vi "plot theory.vi"() -> ()   [LabVIEW 2016]
uses:
  <vilib>/Utility/file.llb/Write Delimited Spreadsheet (DBL).vi
  <userlib>/LevyLab/Graph Utilities/graph_utilities.lvclass
panel:
  in  "color scale":u32[](array[colorbox])=[16711680, 16772608, 6618880, 3381759, 16860, 10420479]
  in  "length 2":i32=200
  in  "index 2":i32
  out "Intensity Graph 13":dbl[][](graph)
  in  "file path (dialog if empty)":path=path "C:/Users/ansom/OneDrive/Pascal Electron Bunching/Figures/Fig 4_new/DMRG stuff/trion_from labview.txt"
  out "Array 2":dbl[][](array[numeric])
  in  "DMRG #":i32=226
  in  "file (use dialog) 4":path=path "C:/Users/ansom/OneDrive/Pascal Electron Bunching/Figures/Fig 4_new/DMRG stuff/trion.txt"
  in  "length":i32=1000
  in  "index":i32
  out "input G":cluster{dbl[], dbl[]}[](graph)
  in  "mu":path=path "C:/Users/ansom/OneDrive/Pascal Electron Bunching/Figures/Fig 3_new/mathematica/mu.txt"
  in  "G":path=path "C:/Users/ansom/OneDrive/Pascal Electron Bunching/Figures/Fig 3_new/mathematica/Gsteps_g=1"
  in  "Numeric 2":i32=100
  in  "Numeric":i32=360
  out "Intensity Graph 12":dbl[][](graph)
  out "Array":dbl[][](array[numeric])
  in  "file (use dialog)":path=path "C:/Users/ansom/OneDrive/Pascal Electron Bunching/Figures/Fig 3_new/mathematica/ModeldGdE"
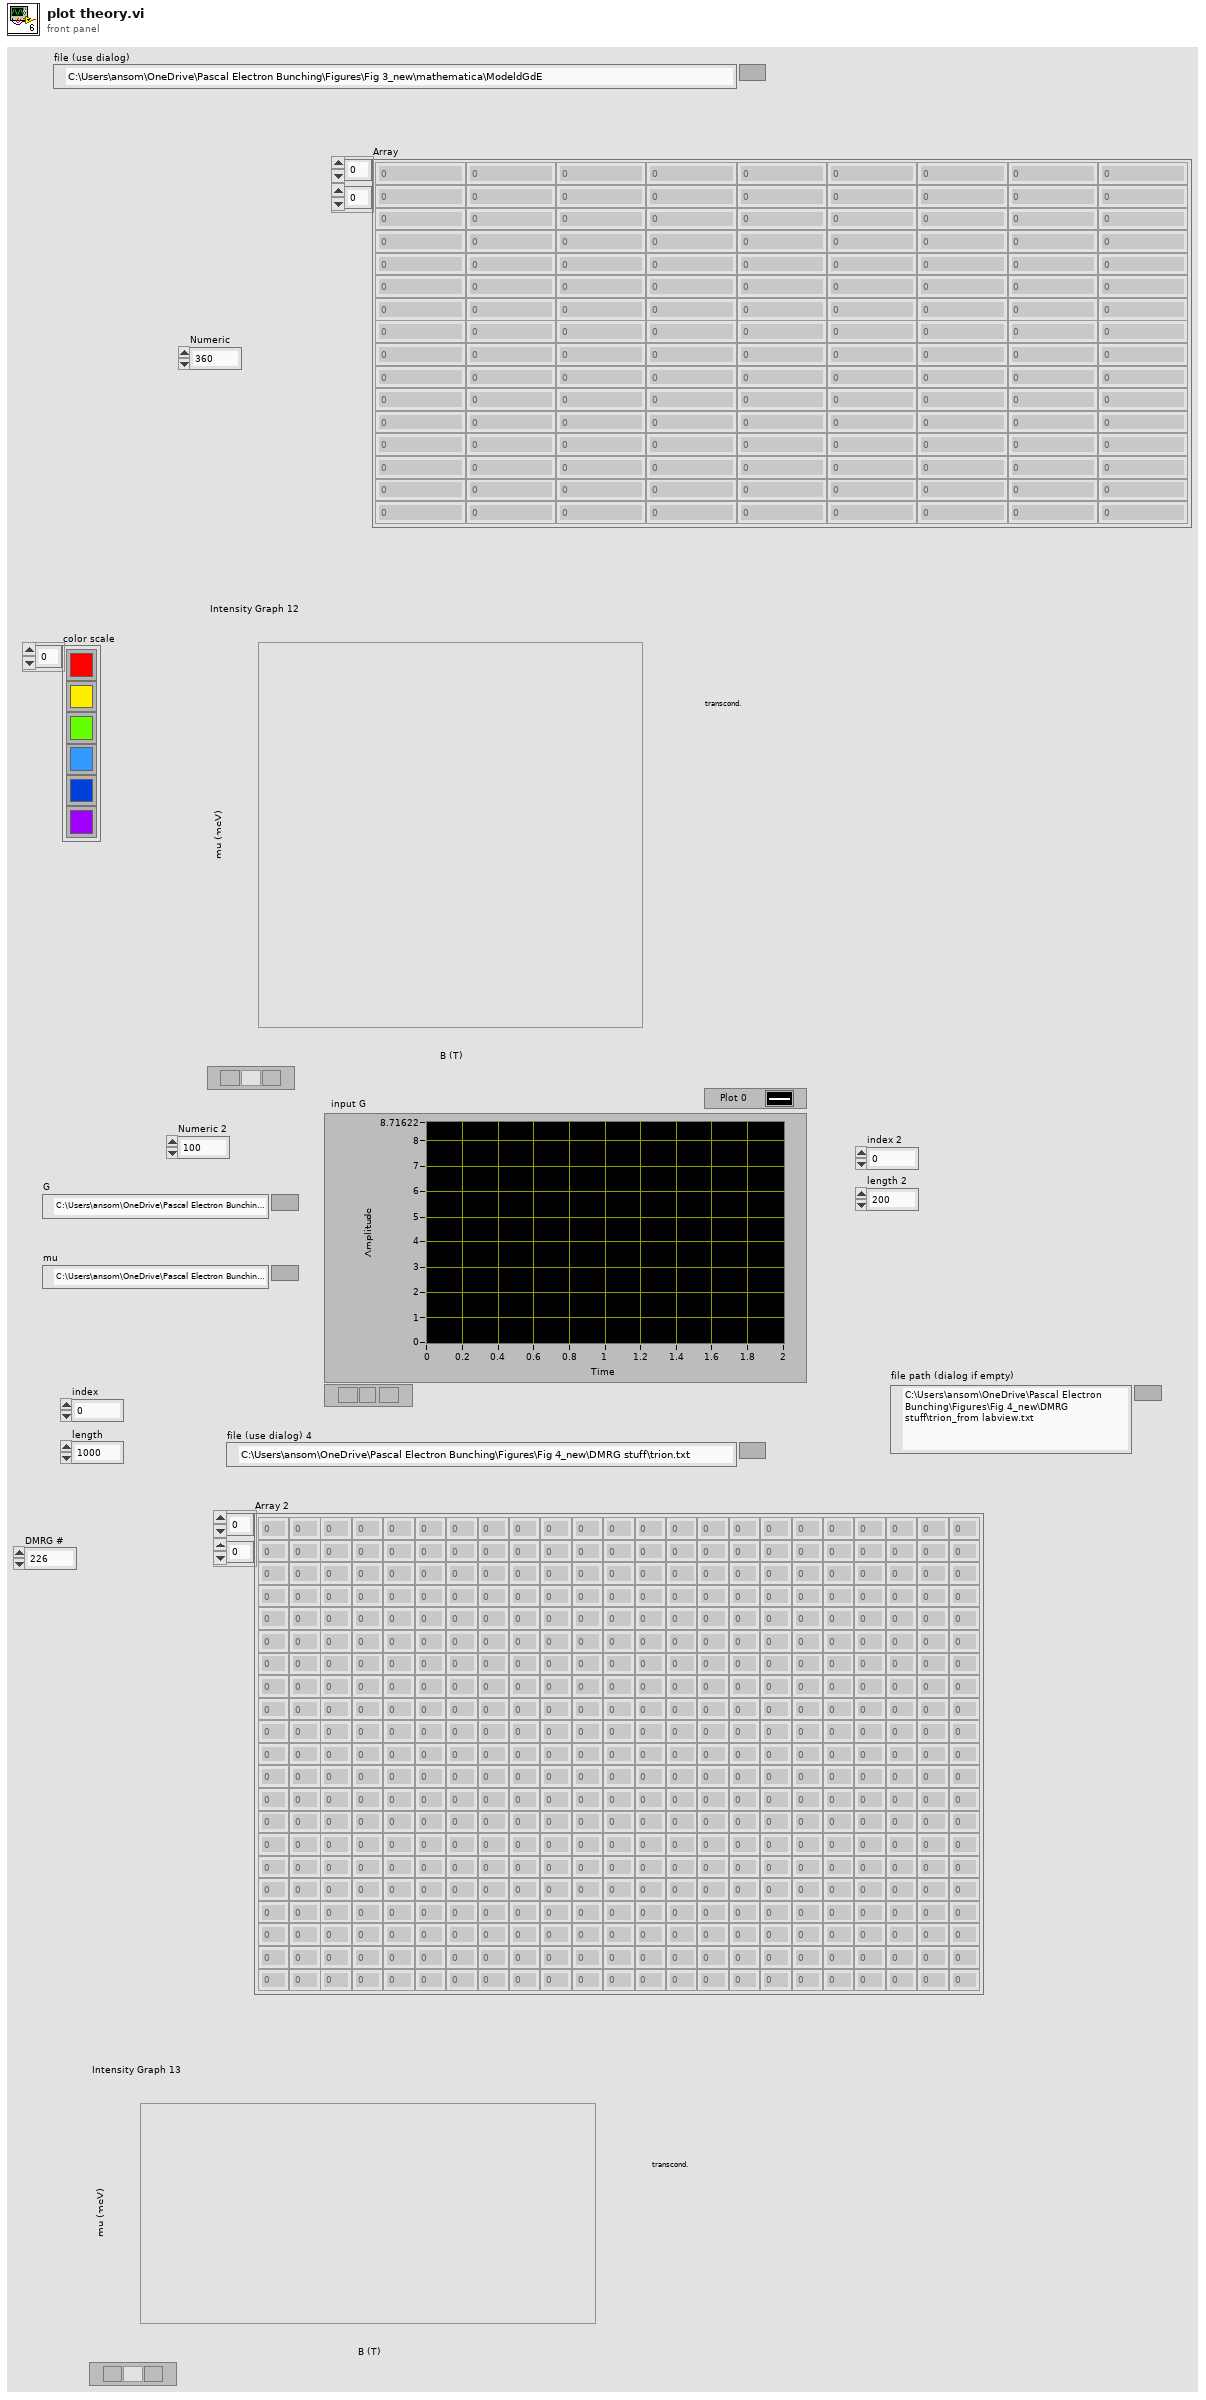
[diagram p1: front panel]
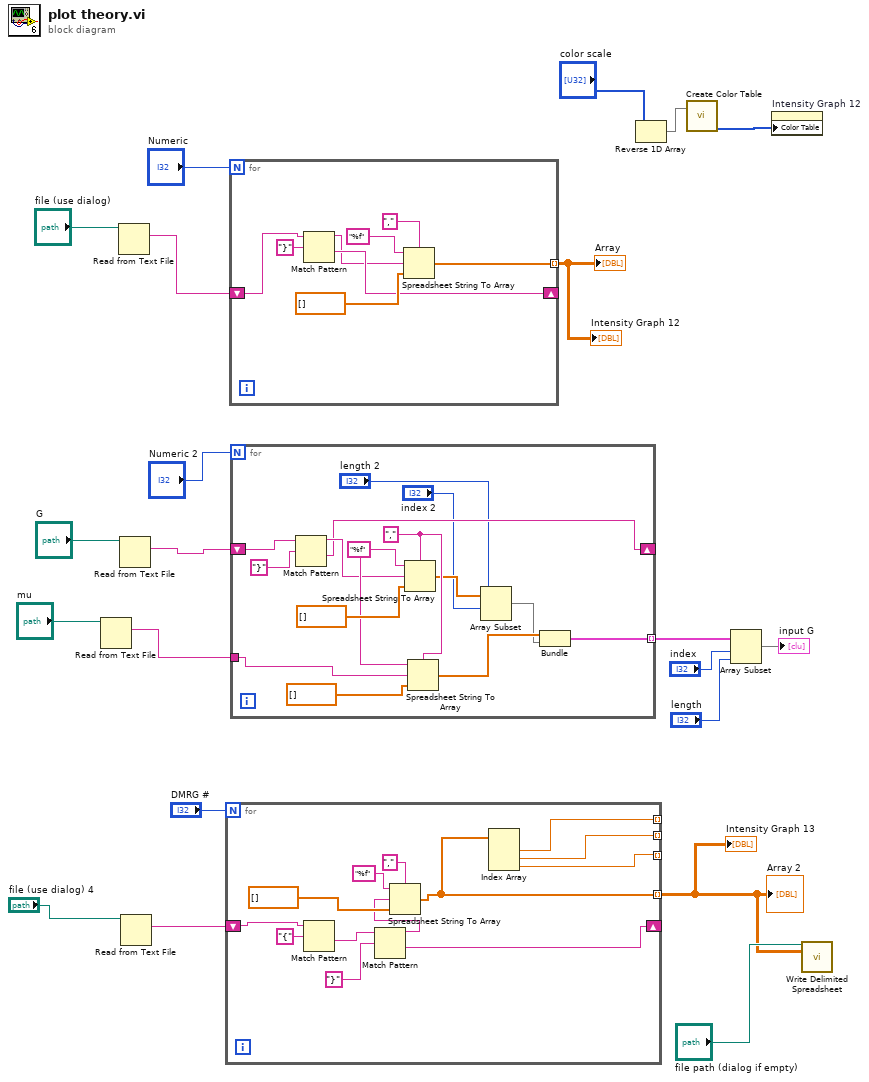
[diagram p0: block diagram]
diagram:
  n1 = Read from Text File(file (use dialog)="mu") -> (text=w14:string)  [unwired: 3 in, 3 out]
  n2 = Read from Text File(file (use dialog)="file (use dialog)") -> (text=w20:string)  [unwired: 3 in, 3 out]
  n3 = Read from Text File(file (use dialog)="G") -> (text=w13:string)  [unwired: 3 in, 3 out]
  n4 = Read from Text File(file (use dialog)="file (use dialog) 4") -> (text=w7:string)  [unwired: 3 in, 3 out]
  n5 = for {
    N: "DMRG #" -> [_]
    shift-right: [w26] -> _
    shift-left: w7 -> [w33]
    tunnel: [w25] -> w4 mode=indexing
    tunnel: [w24] -> _ mode=indexing
    tunnel: [w23] -> _ mode=indexing
    tunnel: [w22] -> _ mode=indexing
    n6 = Match Pattern(string=w33, regular expression="{") -> (after substring=w29:string)  [unwired: 1 in, 3 out]
    n7 = Match Pattern(string=w29, regular expression="}") -> (before substring=w27:string, after substring=w26:string)  [unwired: 1 in, 2 out]
    n8 = Spreadsheet String To Array(delimiter (Tab)=",", format string="%f", spreadsheet string=w27, array type (2D Dbl)=dbl[] []) -> (array=w25:dbl[])
    n9 = Index Array(array=w25) -> (element #1=w24:dbl, element #2=w23:dbl, element #3=w22:dbl)  [unwired: 3 in]
  }
  "Array 2" <- w4
  "Intensity Graph 13" <- w4
  n10 = for {
    N: "Numeric" -> [_]
    tunnel: [w38] -> w18 mode=indexing
    shift-right: [w37] -> _
    shift-left: w20 -> [w36]
    n11 = Match Pattern(string=w36, regular expression="}") -> (before substring=w35:string, after substring=w37:string)  [unwired: 1 in, 2 out]
    n12 = Spreadsheet String To Array(delimiter (Tab)=",", format string="%f", spreadsheet string=w35, array type (2D Dbl)=dbl[] []) -> (array=w38:dbl[])
  }
  "Array" <- w18
  "Intensity Graph 12" <- w18
  n13 = for {
    N: "Numeric 2" -> [_]
    tunnel: w14 -> [w56]
    tunnel: [w52] -> w12 mode=indexing
    shift-right: [w48] -> _
    shift-left: w13 -> [w51]
    w55 = "%f" ("format string")
    w54 = "," ("delimiter (Tab)")
    n14 = Match Pattern(string=w51, regular expression="}") -> (before substring=w49:string, after substring=w48:string)  [unwired: 1 in, 2 out]
    n15 = Spreadsheet String To Array(delimiter (Tab)=w54, format string=w55, spreadsheet string=w49, array type (2D Dbl)=dbl[] []) -> (array=w46:dbl[])
    n16 = Spreadsheet String To Array(delimiter (Tab)=w54, format string=w55, spreadsheet string=w56, array type (2D Dbl)=dbl[] []) -> (array=w47:dbl[])
    n17 = Array Subset(array=w46, index="index 2", length="length 2") -> (w45:dbl[])
    n18 = Bundle(w47, w45) -> (w52:cluster{dbl[], dbl[]})  [unwired: 1 in]
  }
  n19 = Reverse 1D Array(array="color scale") -> (reversed array=w2:u32[])
  n20 = call <userlib>:"Create Color Table.vi"("Colors []"=w2) -> ("Color Tbl"=w3:u32[])  [unwired: 1 in, 3 out]
  n21 = Array Subset(array=w12, index="index", length="length") -> (→"input G":cluster{dbl[], dbl[]}[])
  n22 = property on="Intensity Graph 12" class="IntGraph (strict)"("Color Table"=w3) -> ()  [unwired: 2 in, 2 out]
  n23 = call-poly <vilib>:"Write Delimited Spreadsheet.vi"("file path (dialog if empty)"="file path (dialog if empty)", "2D data"=w4) -> ()  [unwired: 12 in, 2 out]
